vi "WriteUserLog.vi"(1 "Score":i32, 2 "Level":i32, 3 "New User?":bool, 4 "Hashed Password":string, 5 "Username":string, 6 "File Path":path) -> ()   [LabVIEW 2025]
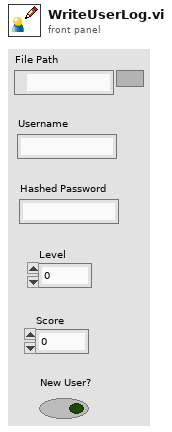
[diagram p1: front panel]
types:
  T1 = enum16{"open", "replace", "create", "open or create", "replace or create", "replace or create with confirmation"}
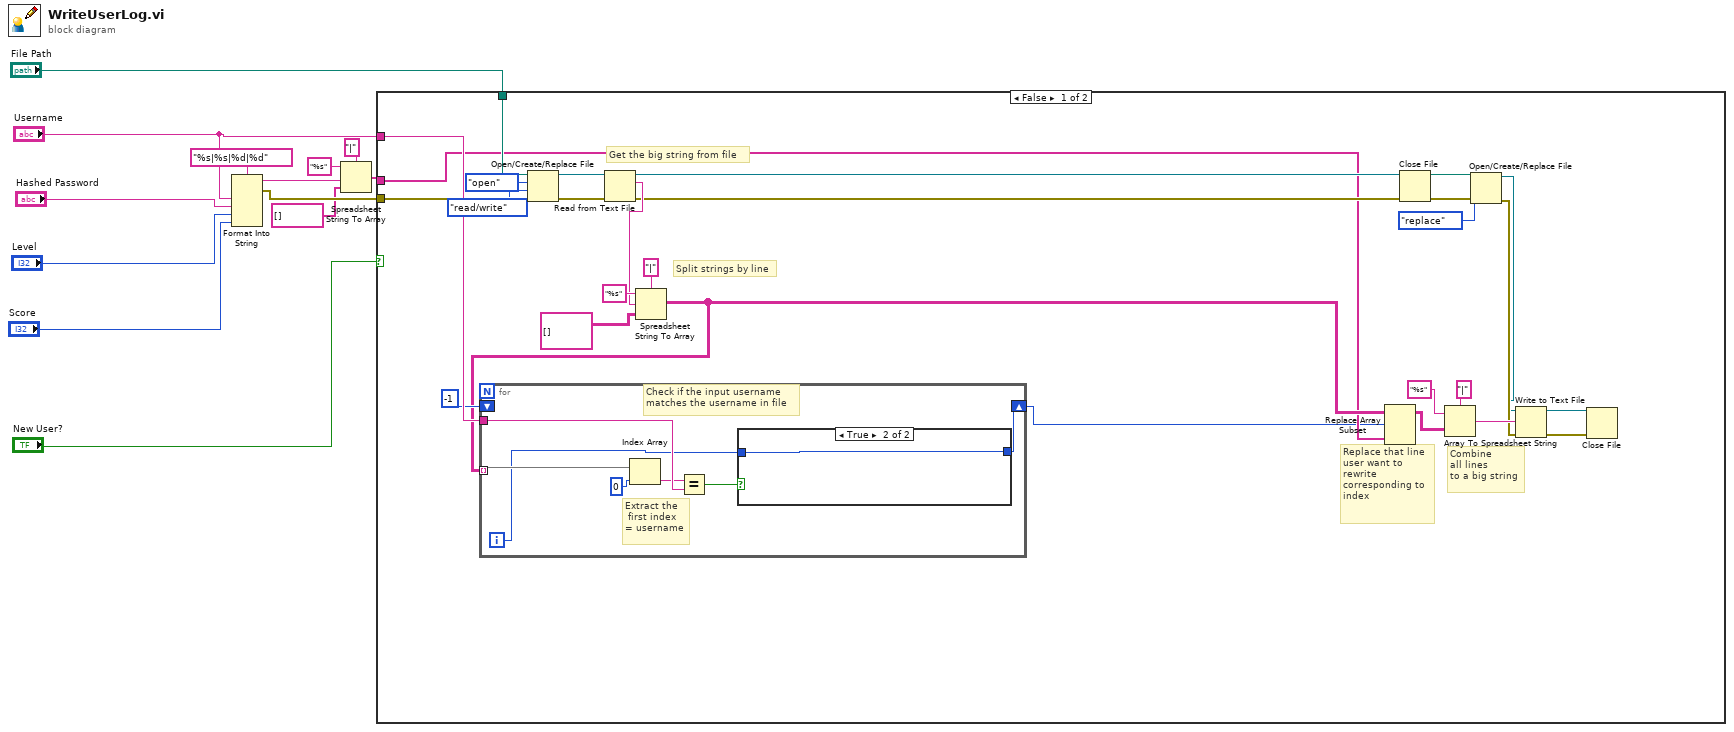
[diagram p0: block diagram]
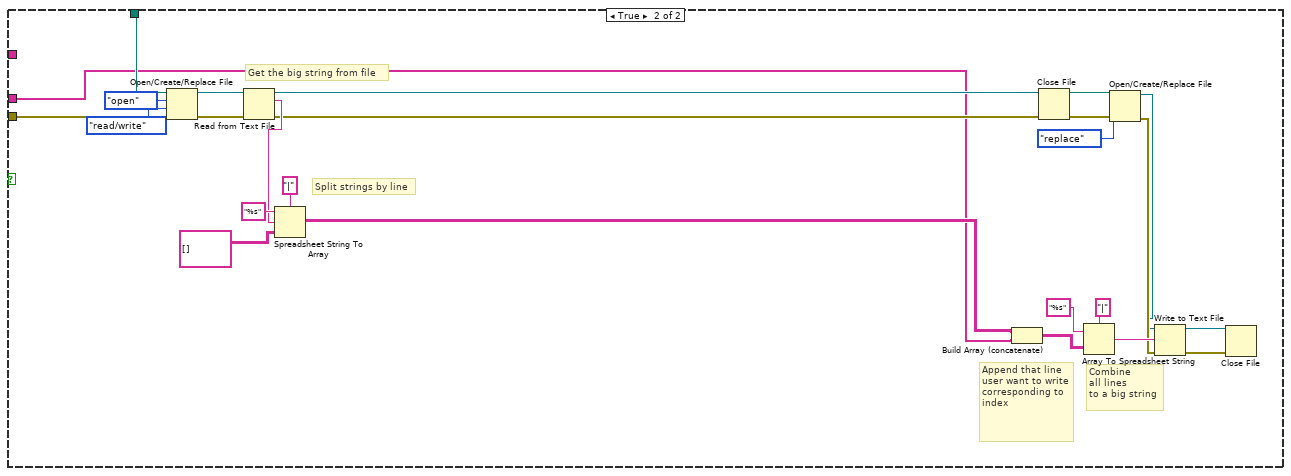
[diagram p3: hidden frame]
diagram:
  n1 = Format Into String(format string="%s|%s|%d|%d", "Username", "Hashed Password", "Level", "Score") -> (resulting string=w5:string, error out=w6:errorcluster)  [unwired: 2 in]
  n2 = Spreadsheet String To Array(delimiter (Tab)="|", format string="%s", spreadsheet string=w5, array type (2D Dbl)=string[] []) -> (array=w3:string[])
  n3 = case shown="False" "New User?" {
    tunnel: "File Path" -> [w41 w54]
    tunnel: w3 -> [w15 w51]
    tunnel: "Username" -> [w36 _]
    tunnel: w6 -> [w26 w53]
    frame False {
      # "Combine \nall lines\nto a big string"
      # "Replace that line \nuser want to rewrite\ncorresponding to index"
      # "Split strings by line"
      # "Get the big string from file"
      n4 = Open/Create/Replace File(file path (use dialog)=w41, error in=w26, operation (0:open)=T1."open", access (0:read/write)=enum16{"read/write", "read-only", "write-only"}."read/write") -> (refnum out=w40:refnum<file>, error out=w39:errorcluster)  [unwired: 2 in, 1 out]
      n5 = Read from Text File(file (use dialog)=w40, error in=w39) -> (refnum out=w22:refnum<file>, text=w34:string, error out=w21:errorcluster)  [unwired: 2 in, 1 out]
      n6 = Spreadsheet String To Array(delimiter (Tab)="|", format string="%s", spreadsheet string=w34, array type (2D Dbl)=string[][] []) -> (array=w33:string[][])
      n7 = for {
        tunnel: w33 -> [w44] mode=indexing
        tunnel: w36 -> [w46]
        shift-right: [w45] -> w14
        shift-left: -1 -> [_]
        i -> [w42]
        # "Check if the input username\nmatches the username in file"
        # "Extract the\n first index \n= username"
        n8 = Index Array(array=w44, index=0) -> (element=w43:string)
        n9 = Equal?(x=w43, y=w46) -> (x = y?=w47:bool)
        n10 = case shown="True" w47 {
          tunnel: [_ w49] -> w45
          tunnel: w42 -> [_ w49]
          frame False {
          }
          frame True {
          }
        }
      }
      n11 = Replace Array Subset(array=w33, new element=w15, index (row)=w14) -> (w32:string[][])  [unwired: 1 in]
      n12 = Close File(refnum=w22, error in=w21) -> (path=w20:path, error out=w19:errorcluster)
      n13 = Array To Spreadsheet String(delimiter (Tab)="|", array=w32, 3:"%s" ("format string")) -> (spreadsheet string=w29:string)
      n14 = Open/Create/Replace File(file path (use dialog)=w20, error in=w19, operation (0:open)=T1."replace") -> (refnum out=w16:refnum<file>, error out=w17:errorcluster)  [unwired: 3 in, 1 out]
      n15 = Write to Text File(file (use dialog)=w16, text=w29, error in=w17) -> (refnum out=w28:refnum<file>, error out=w27:errorcluster)  [unwired: 1 in, 1 out]
      n16 = Close File(refnum=w28, error in=w27) -> ()  [unwired: 2 out]
    }
    frame True {
      # "Combine \nall lines\nto a big string"
      # "Append that line \nuser want to write\ncorresponding to index"
      # "Split strings by line"
      # "Get the big string from file"
      n17 = Open/Create/Replace File(file path (use dialog)=w54, error in=w53, operation (0:open)=T1."open", access (0:read/write)=enum16{"read/write", "read-only", "write-only"}."read/write") -> (refnum out=w74:refnum<file>, error out=w73:errorcluster)  [unwired: 2 in, 1 out]
      n18 = Read from Text File(file (use dialog)=w74, error in=w73) -> (refnum out=w61:refnum<file>, text=w70:string, error out=w60:errorcluster)  [unwired: 2 in, 1 out]
      n19 = Spreadsheet String To Array(delimiter (Tab)="|", format string="%s", spreadsheet string=w70, array type (2D Dbl)=string[][] []) -> (array=w52:string[][])
      n20 = Build Array (concatenate)(w52, w51) -> (w50:string[][])
      n21 = Close File(refnum=w61, error in=w60) -> (path=w59:path, error out=w58:errorcluster)
      n22 = Array To Spreadsheet String(delimiter (Tab)="|", array=w50, 3:"%s" ("format string")) -> (spreadsheet string=w67:string)
      n23 = Open/Create/Replace File(file path (use dialog)=w59, error in=w58, operation (0:open)=T1."replace") -> (refnum out=w55:refnum<file>, error out=w56:errorcluster)  [unwired: 3 in, 1 out]
      n24 = Write to Text File(file (use dialog)=w55, text=w67, error in=w56) -> (refnum out=w66:refnum<file>, error out=w65:errorcluster)  [unwired: 1 in, 1 out]
      n25 = Close File(refnum=w66, error in=w65) -> ()  [unwired: 2 out]
    }
  }
